vi "Driver Init.vi"(8 "error in (no error)":errorcluster, 11 "MSX-E3711 in":refnum<class "MSX-E3711.lvclass">) -> (0 "error out":errorcluster, 3 "MSX-E3711 out":refnum<class "MSX-E3711.lvclass">)   [LabVIEW 2014, in "MSX-E3711.lvlib" / "MSX-E3711.lvclass"]
uses:
  MSX-E3711.lvclass
  MSX-E3711.lvclass/MSX-E3711.ctl
  DriverMasterSync/build/DriverMasterSync.lvlibp/Modules/HAL/DriverMasterSync/DriverMasterSyncClass/DriverMasterSync.lvclass
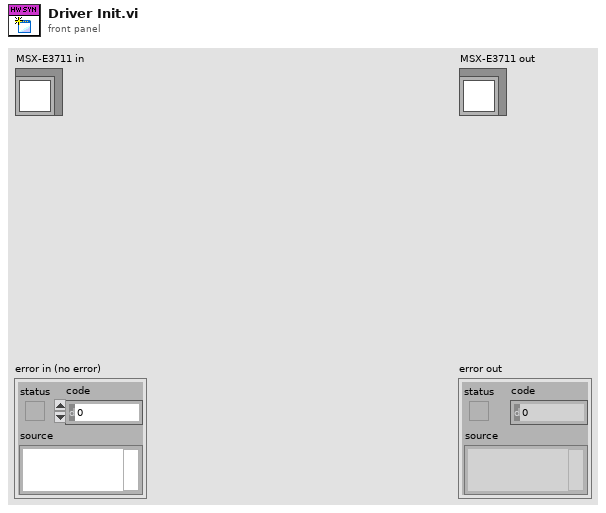
[diagram p1: front panel]
types:
  T1 = typedef "DriverMasterSync.lvlibp/HAL Config Data.ctl" = cluster{"HWSync Index":u32, "Driver Name":string, "Channel Mask":u64}
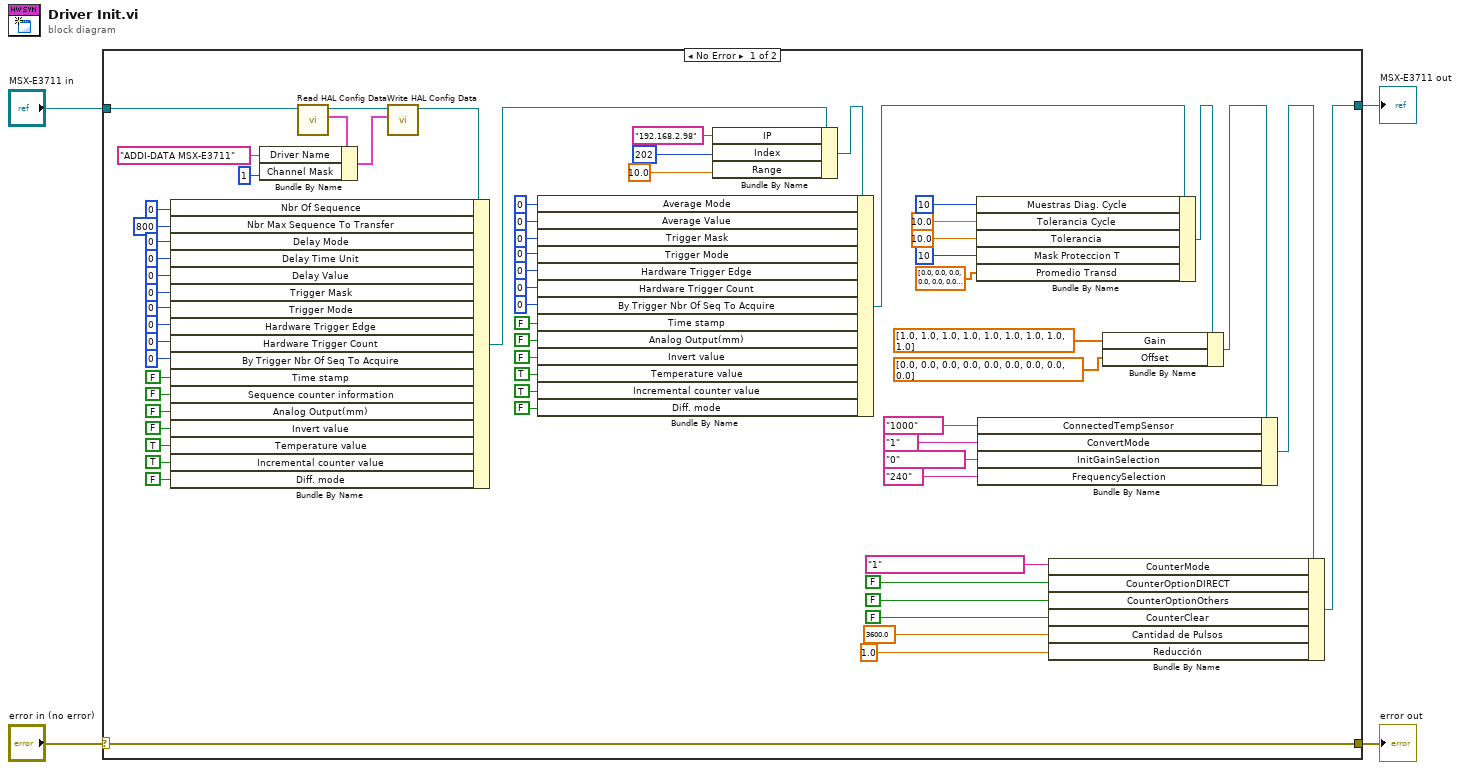
[diagram p0: block diagram]
diagram:
  n1 = case shown="No Error" "error in (no error)" {
    selector: "error in (no error)" -> [w69 w71]
    tunnel: [w69 w71] -> w3
    tunnel: [w15 w70] -> w1
    tunnel: "MSX-E3711 in" -> [w68 w70]
    frame No Error {
      n2 = call "Read HAL Config Data.vi"("DriverMasterSync in"=w68) -> ("HAL Config Data"=w66:T1, "DriverMasterSync out"=w67:refnum<class "MSX-E3711.lvclass">)  [unwired: 8 in, 1 out]
      n3 = Bundle By Name(cluster=w66, "Driver Name"="ADDI-DATA MSX-E3711", "Channel Mask"=u64 1) -> (w65:T1)
      n4 = call "Write HAL Config Data.vi"("HAL Config Data"=w65, "DriverMasterSync in"=w67) -> ("DriverMasterSync out"=w62:refnum<class "MSX-E3711.lvclass">)  [unwired: 8 in, 1 out]
      n5 = Bundle By Name(cluster=w62, "Nbr Of Sequence"=u64 0 ("Config Data.Sequence.Nbr Of Sequence"), "Nbr Max Sequence To Transfer"=u64 800 ("Config Data.Sequence.Nbr Max Sequence To Transfer"), "Delay Mode"=u64 0 ("Config Data.Sequence.Nbr Of Sequence"), "Delay Time Unit"=u64 0 ("Config Data.Sequence.Nbr Max Sequence To Transfer"), "Delay Value"=u64 0 ("Config Data.Sequence.Nbr Of Sequence"), "Trigger Mask"=u64 0 ("Config Data.Sequence.Nbr Max Sequence To Transfer"), "Trigger Mode"=u64 0 ("Config Data.Sequence.Nbr Of Sequence"), "Hardware Trigger Edge"=u64 0 ("Config Data.Sequence.Nbr Max Sequence To Transfer"), "Hardware Trigger Count"=u64 0 ("Config Data.Sequence.Nbr Of Sequence"), "By Trigger Nbr Of Seq To Acquire"=u64 0 ("Config Data.Sequence.Nbr Max Sequence To Transfer"), "Time stamp"=FALSE ("Config Data.Sequence.Time stamp"), "Sequence counter information"=FALSE ("Config Data.Sequence.Sequence counter information"), "Analog Output(mm)"=FALSE ("Config Data.Sequence.Analog Output(mm)"), "Invert value"=FALSE ("Config Data.Sequence.Invert value"), "Temperature value"=TRUE ("Config Data.Sequence.Temperature value"), "Incremental counter value"=TRUE ("Config Data.Sequence.Incremental counter value"), "Diff. mode"=FALSE ("Config Data.Sequence.Diff. mode")) -> (w31:refnum<class "MSX-E3711.lvclass">)
      n6 = Bundle By Name(cluster=w31, "IP"="192.168.2.98" ("Connection Data.IP"), "Index"=u64 202 ("Config Data.Index"), "Range"=sgl 10.0 ("Config Data.Range")) -> (w30:refnum<class "MSX-E3711.lvclass">)
      n7 = Bundle By Name(cluster=w30, "Average Mode"=u64 0 ("Config Data.Sequence.Nbr Max Sequence To Transfer"), "Average Value"=u64 0 ("Config Data.Sequence.Nbr Of Sequence"), "Trigger Mask"=u64 0 ("Config Data.Sequence.Nbr Max Sequence To Transfer"), "Trigger Mode"=u64 0 ("Config Data.Sequence.Nbr Of Sequence"), "Hardware Trigger Edge"=u64 0 ("Config Data.Sequence.Nbr Max Sequence To Transfer"), "Hardware Trigger Count"=u64 0 ("Config Data.Sequence.Nbr Of Sequence"), "By Trigger Nbr Of Seq To Acquire"=u64 0 ("Config Data.Sequence.Nbr Max Sequence To Transfer"), "Time stamp"=FALSE ("Config Data.Sequence.Sequence counter information"), "Analog Output(mm)"=FALSE ("Config Data.Sequence.Analog Output(mm)"), "Invert value"=FALSE ("Config Data.Sequence.Invert value"), "Temperature value"=TRUE ("Config Data.Sequence.Temperature value"), "Incremental counter value"=TRUE ("Config Data.Sequence.Incremental counter value"), "Diff. mode"=FALSE ("Config Data.Sequence.Diff. mode")) -> (w26:refnum<class "MSX-E3711.lvclass">)
      n8 = Bundle By Name(cluster=w26, "Muestras Diag. Cycle"=u32 10 ("Diagnostic Data.Muestras Diag. Cycle"), "Tolerancia Cycle"=sgl 10.0 ("Diagnostic Data.Tolerancia Cycle"), "Tolerancia"=sgl 10.0 ("Diagnostic Data.Tolerancia"), "Mask Proteccion T"=u64 10 ("Diagnostic Data.Mask Proteccion T"), "Promedio Transd"=sgl[] [0.0, 0.0, 0.0, 0.0, 0.0, 0.0, 0.0, 0.0, 0.0, 0.0, 0.0, 0.0, 0.0, 0.0, 0.0, 0.0] ("Diagnostic Data.Promedio Transd")) -> (w20:refnum<class "MSX-E3711.lvclass">)
      n9 = Bundle By Name(cluster=w20, "Gain"=sgl[] [1.0, 1.0, 1.0, 1.0, 1.0, 1.0, 1.0, 1.0, 1.0] ("Config Data.Gain"), "Offset"=sgl[] [0.0, 0.0, 0.0, 0.0, 0.0, 0.0, 0.0, 0.0, 0.0] ("Config Data.Gain")) -> (w17:refnum<class "MSX-E3711.lvclass">)
      n10 = Bundle By Name(cluster=w17, "ConnectedTempSensor"="1000", "ConvertMode"="1", "InitGainSelection"="0", "FrequencySelection"="240") -> (w16:refnum<class "MSX-E3711.lvclass">)
      n11 = Bundle By Name(cluster=w16, "CounterMode"="1", "CounterOptionDIRECT"=FALSE, "CounterOptionOthers"=FALSE, "CounterClear"=FALSE, "Cantidad de Pulsos"=sgl 3600.0 ("Config Data.IncCounter.Cantidad de Pulsos"), "Reducción"=sgl 1.0 ("Config Data.IncCounter.Reducción")) -> (w15:refnum<class "MSX-E3711.lvclass">)
    }
    frame Error {
    }
  }
  "error out" <- w3
  "MSX-E3711 out" <- w1
